vi "createApplication.vi"(8 "error in (no error)":errorcluster, 10 "visibility":i32(ring)=1448165440 items=["Visible"=1448165440, "Invisible"=1448165441], 11 "VGS_RemoteControlClient in":refnum<class "VGS_RemoteControlClient.lvclass">) -> (0 "error out":errorcluster, 3 "VGS_RemoteControlClient out":refnum<class "VGS_RemoteControlClient.lvclass">)   [LabVIEW 2022 SP3, in "LV_VGS.lvlib" / "VGS_RemoteControlClient.lvclass"]
doc: "Creates new VGStudio (MAX) instance remotely. \n\nStarts a new VGStudio (MAX) instance on host Hostname. If call is successful the function returns a valid remote handle and the application state changed from NotRunning to Starting. Afterward, you can poll using getApplicationState() and check when the application has been started.\n\n Currently the application instances per remote computer are limited to one. \n\nParameters\nvisibility defines if VGStudio (MAX) instance is started visibility or not. \n\nReturns\nReturns new RemoteHandle associated with the application instance.\nEmit error RemoteControlServiceIsNotAvailableException if the remote control service doesn't run. \nEmit error UnableToCreateApplicationException if VGStudio (MAX) can't be started. \nEmit error MaximumNumberOfApplicationInstancesIsReachedException if the maximum number of VGStudio (MAX) instances is reached. Currently, it's limited to one instance. \nEmit error GenericLicenseErrorException if no valid VGStudio (MAX) license is present. \nEmit error GenericRemoteControlErrorException if an internal error occurs."
uses:
  VGS_RemoteControlClient.lvclass
  VGS_RemoteControlClient.lvclass/VGS_RemoteControlClient.ctl
  C:/Users/Andrey/Documents/GitHub/LV_VGS/vgs_project.dll
  vgs_project.dll
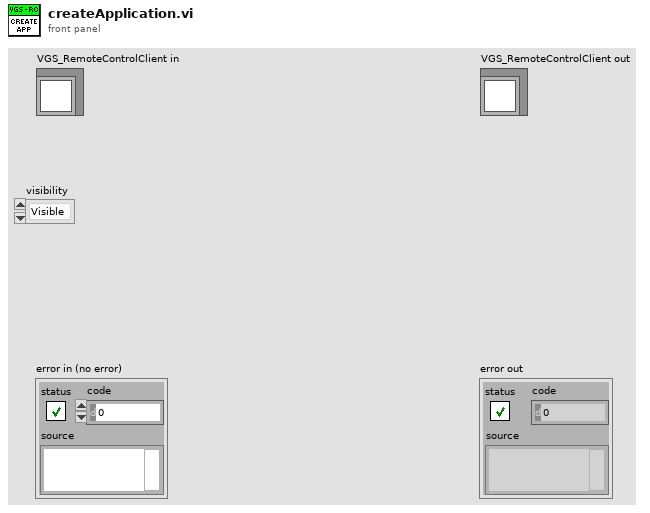
[diagram p1: front panel]
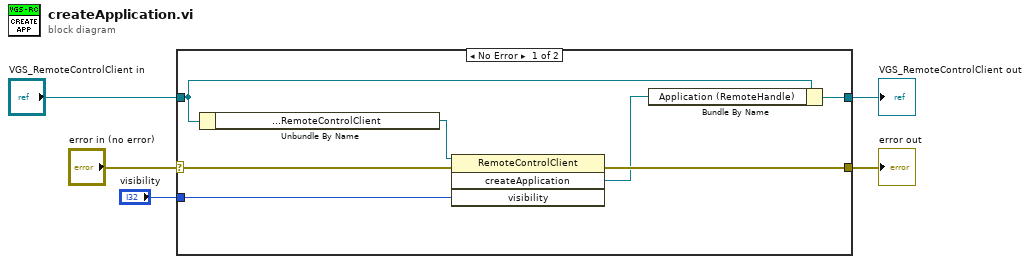
[diagram p0: block diagram]
diagram:
  n1 = case shown="No Error" "error in (no error)" {
    selector: "error in (no error)" -> [w10 w13]
    tunnel: [w9 w13] -> w4
    tunnel: [w12 w14] -> w2
    tunnel: "VGS_RemoteControlClient in" -> [w11 w14]
    tunnel: "visibility" -> [w7 _]
    frame No Error {
      n2 = Unbundle By Name(w11) -> ("VGS.Project.Interop.RemoteControlClient"=w6:refnum<k24>)
      n3 = invoke class="RemoteControlClient" method="createApplication"(reference=w6, error in=w10, "visibility"=w7) -> (error out=w9:errorcluster, "createApplication"=w8:refnum<k24>)  [unwired: 1 in, 2 out]
      n4 = Bundle By Name(cluster=w11, "Application (RemoteHandle)"=w8) -> (w12:refnum<class "VGS_RemoteControlClient.lvclass">)
    }
    frame Error {
    }
  }
  "error out" <- w4
  "VGS_RemoteControlClient out" <- w2
